vi "lookup speed test.vi"() -> ()   [LabVIEW 2013, in "tag bus tests.lvlib"]
uses:
  tag bus tests.lvlib
  dictionary/data dictionary.lvclass
panel:
  out "ok":bool
  out "found":bool[](array[boolean])
  out "x-y":dbl
  in  "count":i32=5000
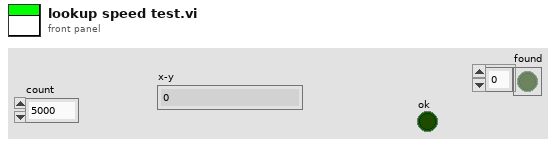
[diagram p1: front panel]
types:
  T1 = typedef "tag bus.lvlib/tag descriptor.lvclass/Data Type.ctl" = enum16{"Double", "Single", "I64", "I32", "I16", "I8", "U64", "U32", "U16", "U8", "Boolean", "String", "Array of Double", "Array of Single", "Array of I64", "Array of I32", "Array of I16", "Array of I8", "Array of U64", "Array of U32", "Array of U16", "Array of U8", "Array of Boolean", "Array of String"}
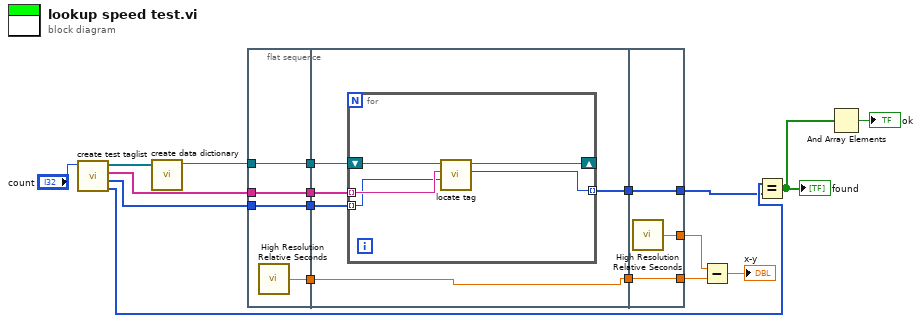
[diagram p0: block diagram]
diagram:
  n1 = call "create test taglist.vi"("count"="count") -> ("indices"=w5:i32[], "types"=w6:T1[], "names/metadata"=w8:string[], "tags"=w17:refnum<class "tag descriptor.lvclass">[])  [unwired: 7 in]
  n2 = call "create data dictionary.vi"("system tags"=w17) -> ("data dictionary"=w10:refnum<class "data dictionary.lvclass">)  [unwired: 9 in, 1 out]
  n3 = flat-sequence {
    tunnel: [w22] -> w13
    tunnel: [w21] -> w11
    tunnel: w10 -> [w21]
    tunnel: [w20] -> w9
    tunnel: w8 -> [w20]
    tunnel: [w19] -> w7
    tunnel: w6 -> [w19]
    tunnel: [w27] -> w15
    tunnel: w13 -> [w27]
    tunnel: w11 -> [w26]
    tunnel: w9 -> [w25]
    tunnel: w7 -> [w24]
    tunnel: [w23] -> w3
    tunnel: [w35] -> w16
    tunnel: w15 -> [w34]
    tunnel: [w34] -> w14
    tunnel: [w33] -> w4
    tunnel: w3 -> [w33]
    frame #0 {
      n4 = call <vilib>:"High Resolution Relative Seconds.vi"() -> ("relative seconds"=w22:dbl)
    }
    frame #1 {
      n5 = for {
        shift-right: [w31] -> _
        shift-left: w26 -> [w32]
        tunnel: w25 -> [w30] mode=indexing
        tunnel: w24 -> [w29] mode=indexing
        tunnel: [w28] -> w23 mode=indexing
        n6 = call "locate tag.vi"("data type"=w29, "name"=w30, "data dictionary in"=w32) -> ("index"=w28:i32, "data dictionary out"=w31:refnum<class "data dictionary.lvclass">)  [unwired: 6 in, 1 out]
      }
    }
    frame #2 {
      n7 = call <vilib>:"High Resolution Relative Seconds.vi"() -> ("relative seconds"=w35:dbl)
    }
  }
  n8 = Subtract(x=w16, y=w14) -> (x-y=→"x-y":dbl)
  n9 = Equal?(x=w5, y=w4) -> (x = y?=w2:bool[])
  "found" <- w2
  n10 = And Array Elements(Boolean array=w2) -> (logical AND=→"ok":bool)
